vi "Delete File.vi"(8 "error in (no error)":errorcluster, 10 "RemoteFileName":string, 11 "FTP in":refnum<class "FTP.lvclass">) -> (0 "error out":errorcluster, 3 "FTP out":refnum<class "FTP.lvclass">)   [LabVIEW 2014, in "FTP.lvlib" / "FTP.lvclass"]
doc: "This vi will delete the file specified by the \"RemoteFileName\" on the FTP Server."
uses:
  FTP.lvclass
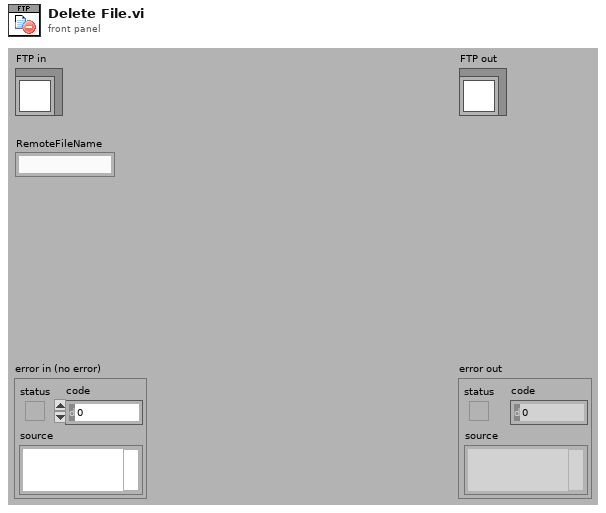
[diagram p1: front panel]
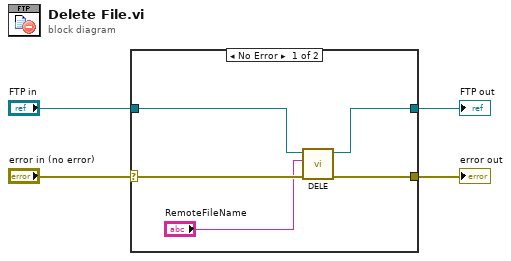
[diagram p0: block diagram]
diagram:
  n1 = case shown="No Error" "error in (no error)" {
    selector: "error in (no error)" -> [w7 w11]
    tunnel: [w6 w11] -> w3
    tunnel: [w8 w10] -> w1
    tunnel: "FTP in" -> [w9 w10]
    frame No Error {
      n2 = call "DELE.vi"("error in (no error)"=w7, "RemoteFileName"="RemoteFileName", "FTP in"=w9) -> ("error out"=w6:errorcluster, "FTP out"=w8:refnum<class "FTP.lvclass">)  [unwired: 7 in]
    }
    frame Error {
    }
  }
  "error out" <- w3
  "FTP out" <- w1
